vi "Custom Data.vi"() -> (0 "ErrOut":errorcluster)   [LabVIEW 2016]
doc: "Use this template to build a VI to use as a subVI."
uses:
  <vilib>/vision/Image Controls.llb/Vision Info Type2.ctl
  <vilib>/vision/NI_Vision_Development_Module.lvlib
panel:
  out "Present?":bool=TRUE
  out "Keys":string[](array[string])
  out "Custom Data Out":string
  in  "ErrIn":errorcluster
  # "Input Parameters"
  # "Output Parameters"
  # "VI Description:\nThis VI is .."
  # ":: MVI Framework V1.0 ::\nAuthor:Gaoke Yang\nEmail: gaoke.yang@yahoo.com\nWeb: www.mvicontrol.com\nCopyright (C) 2013, MVI Technologies All Rights Reserved"
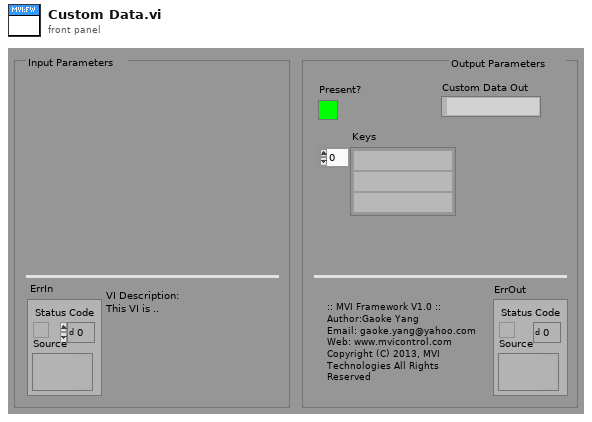
[diagram p1: front panel]
types:
  T1 = typedef "Vision Info Type2.ctl" = u32
  T2 = typedef "Image Type" = u32
  T3 = typedef "IMAQ Image.ctl" = refnum<image>
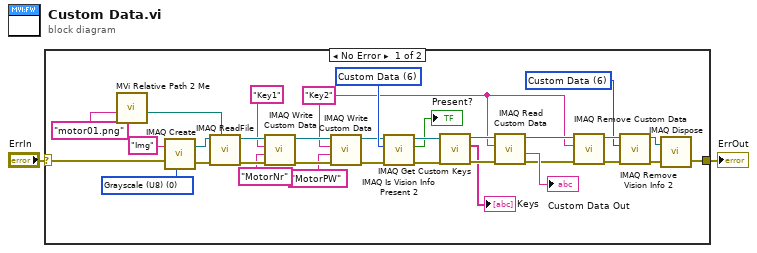
[diagram p0: block diagram]
diagram:
  n1 = case shown="No Error" "ErrIn" {
    selector: "ErrIn" -> [w22 w36]
    tunnel: [w32 w36] -> w2
    frame No Error {
      w5 = T1 6 items=["Any", "Calibration", "Overlay", "Grayscale Template", "Color Template", "Geometric Template", "Custom Data", "Golden Template", "Geometric Template 2", "Contour Data", "Camera Model", "Pyramid Grayvalue Template", "Pyramid Gradient Template"] ("Vision Info")
      w10 = "Key2" ("Key")
      w30 = T2 0 items=["Grayscale (U8)", "Grayscale (I16)", "Grayscale (SGL)", "Complex (CSG)", "RGB (U32)", "HSL (U32)", "RGB (U64)", "Grayscale (U16)"] ("Image Type")
      w31 = T1 6 items=["Any", "Calibration", "Overlay", "Grayscale Template", "Color Template", "Geometric Template", "Custom Data", "Golden Template", "Geometric Template 2", "Contour Data", "Camera Model", "Pyramid Grayvalue Template", "Pyramid Gradient Template"] ("Vision Info")
      n2 = call "MVi Relative Path 2 Me.vi"("Relative Path"="motor01.png" ("name or relative path")) -> ("Appended Dir"=w3:path)  [unwired: 5 in, 1 out]
      n3 = call "IMAQ Create"("Image Name"="Img", "Image Type"=w30, "error in (no error)"=w22) -> ("New Image"=w34:T3, "error out"=w33:errorcluster)  [unwired: 2 in]
      n4 = call "IMAQ ReadFile"("File Path"=w3, "error in (no error)"=w33, "Image"=w34) -> ("error out"=w28:errorcluster, "Image Out"=w29:T3)  [unwired: 4 in, 3 out]
      n5 = call "IMAQ Write Custom Data"("error in (no error)"=w28, "Custom Data In"="MotorNr", "Key"="Key1", "Image"=w29) -> ("error out"=w15:errorcluster, "Image Out"=w14:T3)  [unwired: 6 in]
      n6 = call "IMAQ Write Custom Data"("error in (no error)"=w15, "Custom Data In"="MotorPW", "Key"=w10, "Image"=w14) -> ("error out"=w11:errorcluster, "Image Out"=w12:T3)  [unwired: 6 in]
      n7 = call "IMAQ Is Vision Info Present 2"("error in (no error)"=w11, "Vision Info"=w31, "Image"=w12) -> ("error out"=w23:errorcluster, "Present?"=→"Present?":bool, "Image (duplicate)"=w24:T3)  [unwired: 6 in]
      n8 = call "IMAQ Get Custom Keys"("error in (no error)"=w23, "Image"=w24) -> ("error out"=w26:errorcluster, "Keys"=→"Keys":string[], "Image (duplicate)"=w25:T3)  [unwired: 6 in, 1 out]
      n9 = call "IMAQ Read Custom Data"("error in (no error)"=w26, "Key"=w10, "Image"=w25) -> ("error out"=w18:errorcluster, "Custom Data Out"=→"Custom Data Out":string, "Image (duplicate)"=w17:T3)  [unwired: 6 in]
      n10 = call "IMAQ Remove Custom Data"("error in (no error)"=w18, "Key"=w10, "Image"=w17) -> ("error out"=w7:errorcluster, "Image Out"=w6:T3)  [unwired: 6 in, 1 out]
      n11 = call "IMAQ Remove Vision Info 2"("error in (no error)"=w7, "Vision Info"=w5, "Image"=w6) -> ("error out"=w9:errorcluster, "Image Out"=w8:T3)  [unwired: 7 in]
      n12 = call "IMAQ Dispose"("Image"=w8, "error in (no error)"=w9) -> ("error out"=w32:errorcluster)  [unwired: 4 in]
    }
    frame Error {
    }
  }
  "ErrOut" <- w2
